vi "Get Duty Cycle.vi"(7 "Channel (1: Chan A)":i32(ring)=1 items=["System (To)", "Channel A", "Channel B", "Channel C", "Channel D", "Channel E", "Channel F", "Channel G", "Channel H"], 8 "error in (no error)":errorcluster, 11 "VISA resource name":refnum<visa-resource-name>) -> (0 "error out":errorcluster, 1 "DC Off":i32=-1, 2 "DC On":i32=-1, 3 "VISA resource name out":refnum<visa-resource-name>)   [LabVIEW 2013, in "Berkeley Nucleonics 500 Series.lvlib"]
doc: "This VI is used to read the duty cycle configuration of the selected channel or system timer (To)."
uses:
  Berkeley Nucleonics 500 Series.lvlib
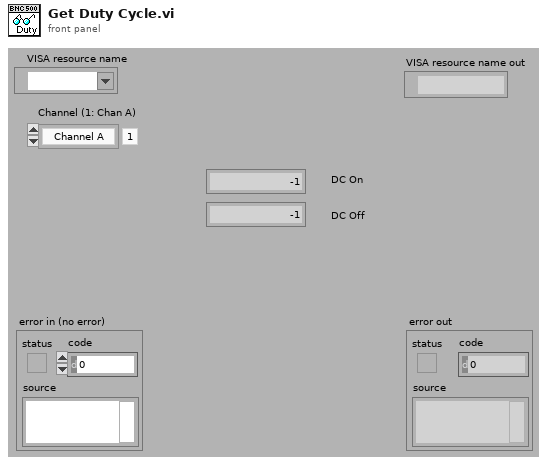
[diagram p1: front panel]
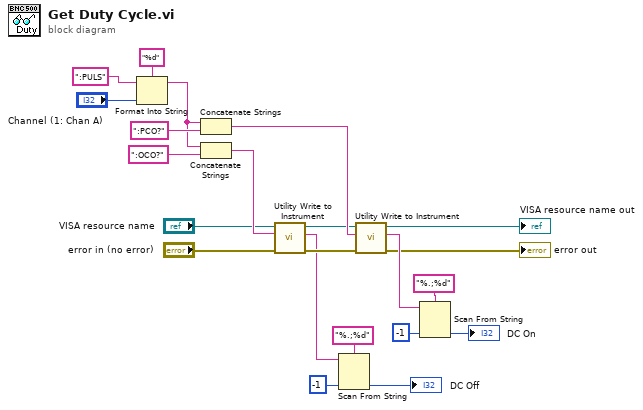
[diagram p0: block diagram]
diagram:
  n1 = Format Into String(format string="%d", initial string=":PULS", "Channel (1: Chan A)") -> (resulting string=w1:string)  [unwired: 1 in, 1 out]
  n2 = Concatenate Strings(w1, ":PCO?") -> (w16:string)
  n3 = Concatenate Strings(w1, ":OCO?") -> (w14:string)
  n4 = call "Utility Write to Instrument.vi"("error in (no error)"="error in (no error)", "Write Buffer"=w14, "VISA resource name"="VISA resource name") -> ("error out"=w13:errorcluster, "Read Buffer"=w9:string, "VISA resource name out"=w12:refnum<visa-resource-name>)  [unwired: 6 in]
  n5 = Scan From String(format string="%.;%d", input string=w9, default 1=-1 ("default value 1")) -> (output 1=→"DC Off":i32)  [unwired: 2 in, 3 out]
  n6 = call "Utility Write to Instrument.vi"("error in (no error)"=w13, "Write Buffer"=w16, "VISA resource name"=w12) -> ("error out"=→"error out":errorcluster, "Read Buffer"=w18:string, "VISA resource name out"=→"VISA resource name out":refnum<visa-resource-name>)  [unwired: 6 in]
  n7 = Scan From String(format string="%.;%d", input string=w18, default 1=-1 ("default value 1")) -> (output 1=→"DC On":i32)  [unwired: 2 in, 3 out]
